vi "Sensor data visualisation.vi"() -> ()   [LabVIEW 2014]
uses:
  <vilib>/LVH/AR Drone Toolkit/Decode NavData/Typedefs/NavData Demo.ctl
  <vilib>/Native 3D Graph/xcontrol/3DPC_SurfacePlot.xctl
  <vilib>/Native 3D Graph/classes/Line/Line.lvclass
  <vilib>/LVH/AR Drone Toolkit/AR Drone.lvlib
panel:
  in  "Emergency Landing":bool
  in  "Switch control":bool=TRUE
  in  "Tab Control 2":enum32{"Altitude", "Tilt sensor", "Speed data"}(tab)
  out "Altitude":u32(graph)
  out "Tilt":T1(graph)={"pitch (deg)"=0.068, "roll (deg)"=-0.016, "yaw (deg)"=0.828}
  out "vy":sgl(graph)
  out "vx":sgl(graph)
  in  "Tab Control":enum32{"2D Position", "3D Position"}(tab)
  out "XY Graph":cluster{"Y":dbl[], "Y":dbl[]}[](graph)
  out "3D Graph":refnum<class "Base Datatype.lvclass">[](xcontrol)
  out "Battery Remaining":dbl(slide)=97.0 scale=0.0..100.0
  out "NavData Out":T2={"control state"=enum."TRANS_LANDING", "battery percentage"=97, "pitch (deg)"=0.068, "roll (deg)"=-0.016, "yaw (deg)"=0.828, "altitude (cm)"=0, "vx (cm/s)?"=0.0, "vy (cm/s)?"=0.0, "vz (cm/s)?"=0.0, "detection cam type"=3}
  out "nav":errorcluster
  out "ctr":errorcluster
  in  "stop":bool
  # "1. The initial position is set to (0,0).\n\n2. The next position is calculated based exclusively on the incoming sensor data (dispalyed in the Speed data tab below).\n\n3. The last 1000 coordinates are stored in an array and are displayed on an XY Graph."
  # "Here we use the same principles as in the 2D Position, but we also add the Altitude sensor data as the third dimension.\n\n1 unit equals 1 mm."
  # "Double-click the Plot to open it in a separate, bigger window."
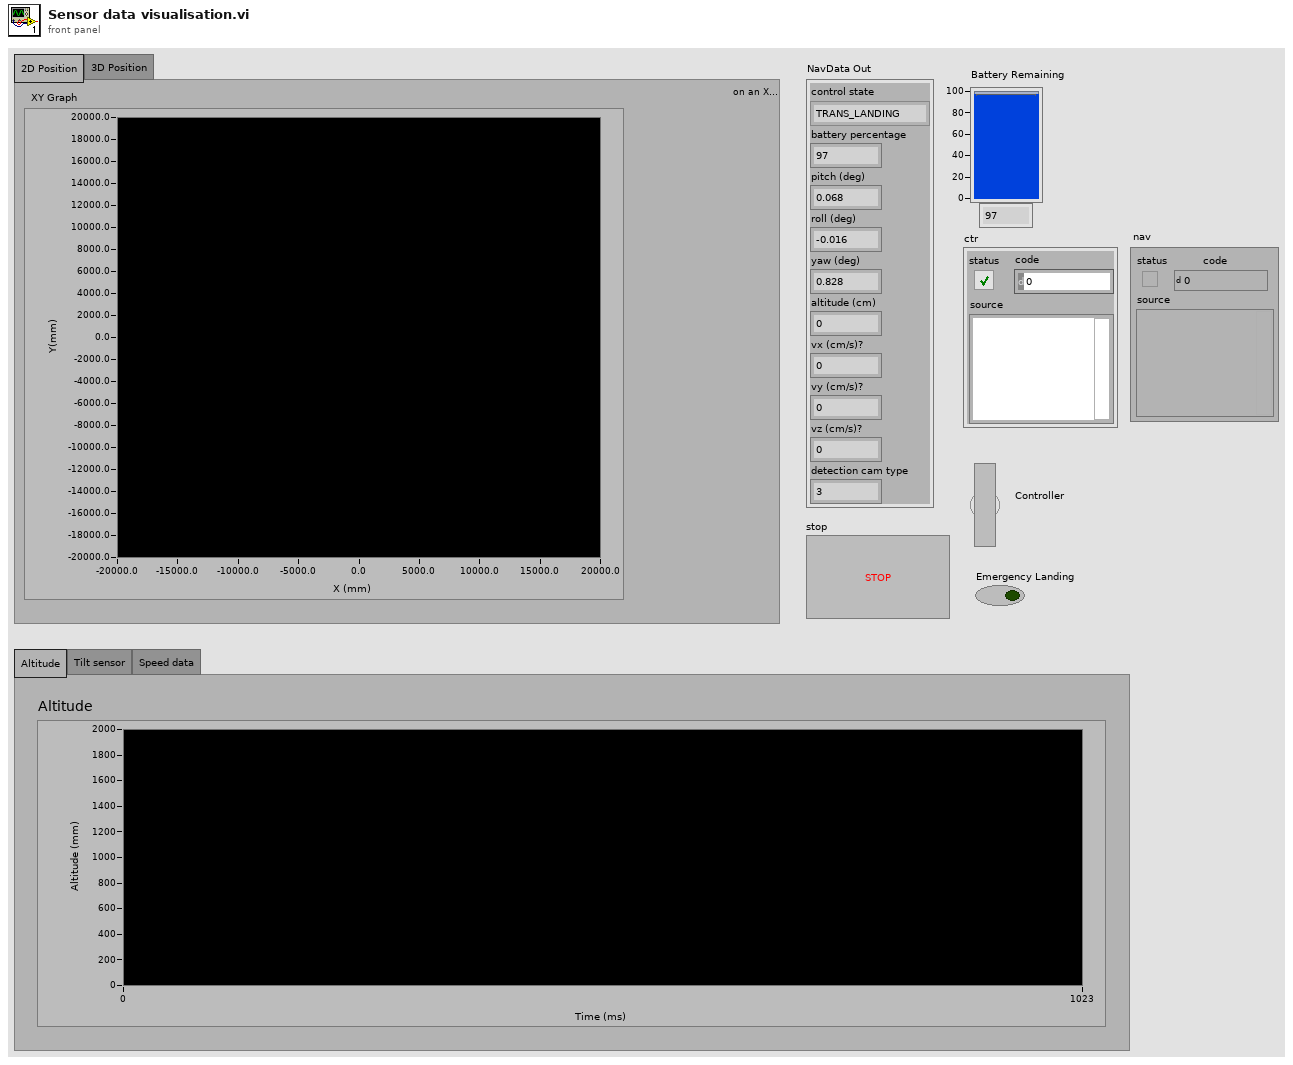
[diagram p1: front panel]
types:
  T1 = cluster{"pitch (deg)":sgl, "roll (deg)":sgl, "yaw (deg)":sgl}
  T2 = typedef "AR Drone.lvlib/NavData Demo.ctl" = cluster{"control state":enum32{"DEFAULT", "INIT", "LANDING", "FLYING", "HOVERING", "TEST", "TRANS_TAKEOFF", "TRANS_GOTOFIX", "TRANS_LANDING"}, "battery percentage":u32, "pitch (deg)":sgl, "roll (deg)":sgl, "yaw (deg)":sgl, "altitude (cm)":u32, "vx (cm/s)?":sgl, "vy (cm/s)?":sgl, "vz (cm/s)?":sgl, "detection cam type":u32}
  T3 = typedef "AR Drone.lvlib/AR Drone Resource.ctl" = cluster{"UDP Control Connection":refnum<k16>, "UDP NavData Connection":refnum<k16>, "UDP Video Connection (Drone 1.0)":refnum<k16>, "TCP Video Connection (Drone 2.0)":refnum<k5>, "TCP Control Port Connection":refnum<k5>, "Drone IP address":string, "Drone Command Port":u16, "Drone NavData Port":u16, "Drone Vid Stream Port":u16, "Drone TCP Control Port":u16, "Home IP address":string, "Home Command Port":u16, "Home NavData Port":u16, "Home Vid Stream Port":u16, "Drone Version":i32, "Drone Index":i32, "Command Sequence":i32}
  T4 = cluster{"Roll":dbl, "Pitch":dbl, "Vertical Speed":dbl, "Yaw Speed":dbl}
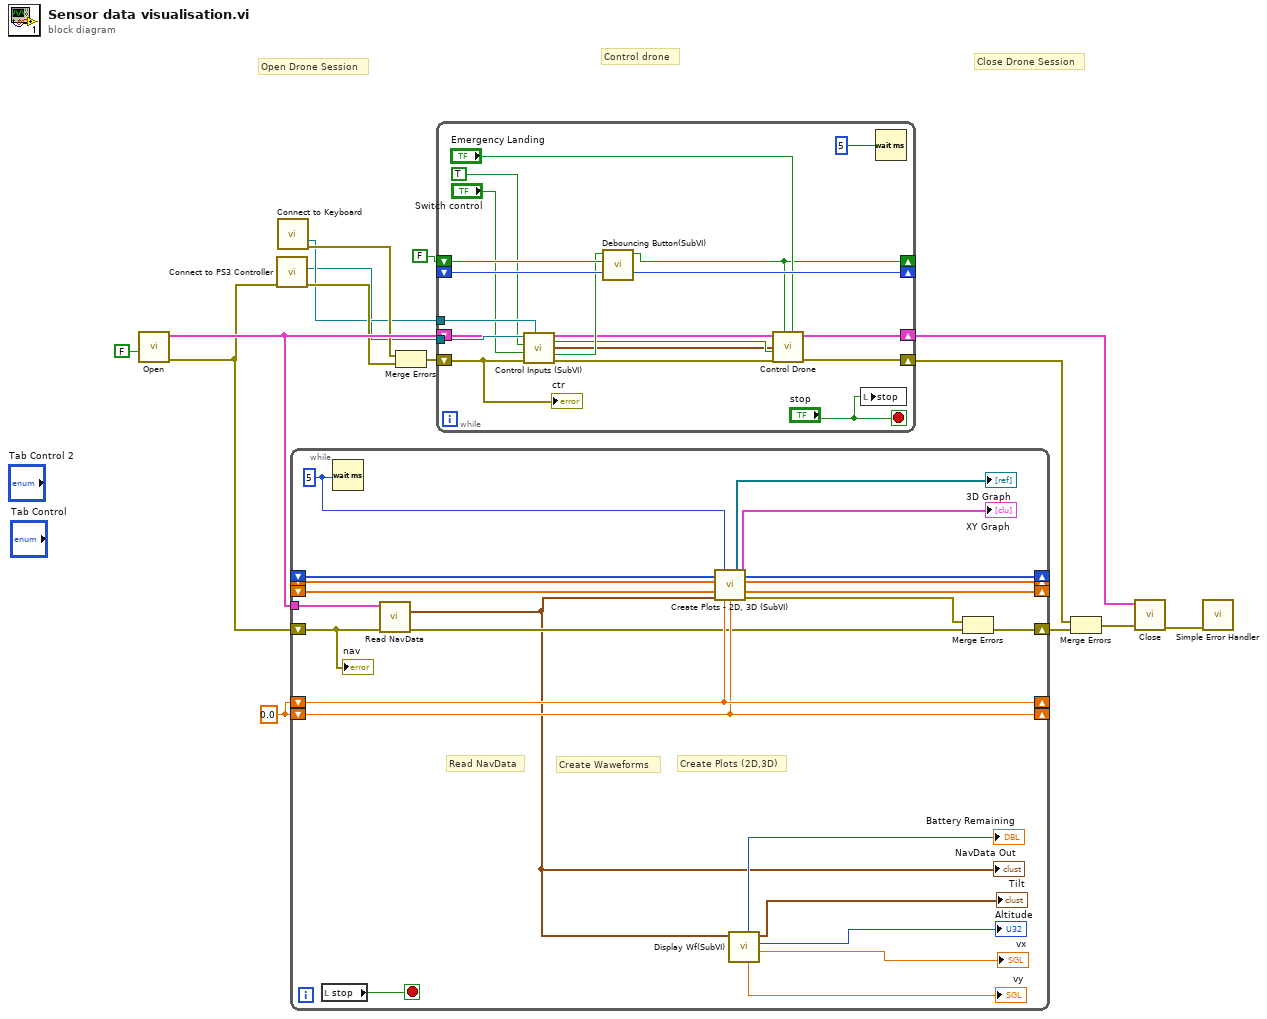
[diagram p0: block diagram]
diagram:
  w11 = 0.0
  # "Control drone"
  # "Close Drone Session"
  # "Open Drone Session"
  n1 = call <vilib>:"Open.vi"("Init Video?"=FALSE) -> ("error out"=w7:errorcluster, "AR Drone Resource"=w8:T3)  [unwired: 9 in]
  n2 = call "Connect to PS3 Controller.vi"("error in (no error)"=w7) -> ("error out"=w5:errorcluster, "device ID 2"=w1:refnum<k1>)  [unwired: 8 in]
  n3 = call "Connect to Keyboard.vi"() -> ("device ID"=w2:refnum<k1>, "error out"=w4:errorcluster)  [unwired: 13 in, 1 out]
  n4 = while {
    shift-right: [w18] -> w12
    shift-left: w7 -> [w17]
    shift-right: [w34] -> _
    shift-left: _ -> [w25]
    shift-right: [w33] -> _
    shift-left: _ -> [w36]
    shift-right: [w22] -> _
    shift-left: w11 -> [w22]
    shift-right: [w23] -> _
    shift-left: w11 -> [w23]
    shift-right: [w31] -> _
    shift-left: _ -> [w32]
    tunnel: w8 -> [w37]
    stop <- w38 stop-if-true
    w24 = u32 5 ("milliseconds to wait")
    # "Create Waweforms"
    # "Create Plots (2D,3D)"
    # "Read NavData"
    n5 = local read "stop"() -> (w38:bool)
    n6 = Wait (ms)(milliseconds to wait=w24) -> ()  [unwired: 1 out]
    n7 = call <vilib>:"Read NavData.vi"("error in (no error)"=w17, "AR Drone Resource"=w37) -> ("error out"=w20:errorcluster, "NavData Out"=w16:T2)  [unwired: 7 in, 1 out]
    "NavData Out" <- w16
    n8 = call "Create Plots - 2D, 3D (SubVI).vi"("Array in"=w32, "milliseconds to wait"=w24, "X array in"=w25, "Y array in"=w36, "NavData Out"=w16, "Numeric 2"=w23, "Numeric"=w22) -> ("3D Graph"=→"3D Graph":refnum<class "Base Datatype.lvclass">[], "XY Graph"=→"XY Graph":cluster{"Y":dbl[], "Y":dbl[]}[], "Array out"=w31:u32[], "X array out"=w34:dbl[], "Y array out"=w33:dbl[], "error out"=w21:errorcluster)  [unwired: 3 in]
    n9 = call "Display Wf(SubVI).vi"("NavData Out"=w16) -> ("vx (cm/s)?"=→"vx":sgl, "altitude (cm)"=→"Altitude":u32, "Cluster"=→"Tilt":T1, "vy (cm/s)?"=→"vy":sgl, "battery percentage"=→"Battery Remaining":u32)  [unwired: 6 in]
    n10 = Merge Errors(w21, w20) -> (w18:errorcluster)
    "nav" <- w17
  }
  n11 = Merge Errors(w4, w5) -> (w6:errorcluster)
  n12 = while {
    shift-right: [w57] -> w15
    shift-left: w8 -> [w39]
    shift-right: [w40] -> w13
    shift-left: w6 -> [w47]
    shift-right: [w42] -> _
    shift-left: FALSE ("Boolean out") -> [w55]
    shift-right: [w54] -> _
    shift-left: _ -> [w53]
    tunnel: w2 -> [w51]
    tunnel: w1 -> [w50]
    stop <- "stop" stop-if-true
    n13 = call "Control Inputs (SubVI).vi"("Keyboard ID"=w51, "error in (no error)"=w47, "Switch control"="Switch control", "Manual"=TRUE, "Controller ID"=w50) -> ("error out"=w41:errorcluster, "Land/Take off"=w46:bool, "Boolean"=w45:bool, "Control cluster"=w44:T4)  [unwired: 3 in]
    n14 = call "Debouncing Button(SubVI).vi"("millisecond timer value in"=w53, "Boolean in"=w55, "Land/Take off"=w46) -> ("millisecond timer value out"=w54:u32, "Boolean out"=w42:bool)  [unwired: 7 in]
    n15 = call <vilib>:"Control Drone.vi"("Emergency Landing"="Emergency Landing", "Takeoff/Land"=w42, "error in (no error)"=w41, "Hover"=w45, "Control Cluster"=w44, "AR Drone Resource"=w39) -> ("error out"=w40:errorcluster, "AR Drone Resource Out"=w57:T3)  [unwired: 4 in]
    n16 = local write "stop"("stop") -> ()
    n17 = Wait (ms)(milliseconds to wait=u32 5) -> ()  [unwired: 1 out]
    "ctr" <- w47
  }
  n18 = Merge Errors(w13, w12) -> (w9:errorcluster)
  n19 = call <vilib>:"Close.vi"("error in (no error)"=w9, "AR Drone Resource"=w15) -> ("error out"=w14:errorcluster)  [unwired: 9 in]
  n20 = call <vilib>:"Simple Error Handler.vi"("error in (no error)"=w14) -> ()  [unwired: 4 in, 5 out]
